vi "Test function.vi"(11 "Array":dbl[](array[numeric])) -> (3 "Error":dbl)   [LabVIEW 2016]
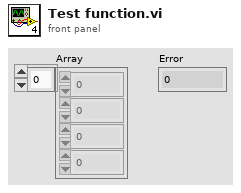
[diagram p1: front panel]
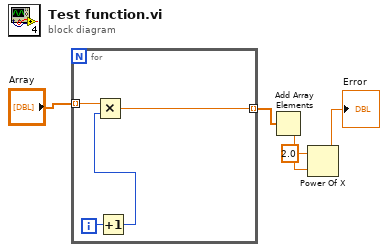
[diagram p0: block diagram]
diagram:
  n1 = for {
    tunnel: "Array" -> [w9] mode=indexing
    tunnel: [w6] -> w4 mode=indexing
    i -> [w7]
    n2 = Increment(x=w7) -> (x+1=w8:i32)
    n3 = Multiply(x=w9, y=w8) -> (x*y=w6:dbl)
  }
  n4 = Add Array Elements(numeric array=w4) -> (sum=w3:dbl)
  n5 = Power Of X(1:w3, 2:2.0 ("y")) -> (0:→"Error":dbl)
